vi "PhotonCamera_TakeOutputSnapshot.vi"(9 "BaseNTName":string="/photonvision", 11 "CameraName":string) -> (0 "error out":errorcluster)   [LabVIEW 2019, in "PhotonVisionLib.lvlib"]
doc: "Request the camera to save a new image file from the output stream with overlays. Images take up space in the filesystem of the PhotonCamera. Calling it frequently will fill up disk space and eventually cause the system to stop working. Clear out images in /opt/photonvision/photonvision_config/imgSaves frequently to prevent issues.\n\nInputs:\n - CameraName -- The nickname of the camera (found in the PhotonVision UI).\n - BaseNTName - string - Base Nework Table name. (Optional. Default: /photonvision )\n\nOutputs:\n - Error Out -- Contains error information if a Network table ot other error occured."
uses:
  PhotonVisionLib.lvlib
  <vilib>/Rock Robotics/WPI/ThirdParty/JAS_Junk/TrajLib/VI/Util_GetTime_U32.vi
  <vilib>/Rock Robotics/WPI/ThirdParty/JAS_Junk/TrajLib/VI/Util_GetTime_U64.vi
  <vilib>/Rock Robotics/Network Tables/NT Read Integer.vi
  <vilib>/Rock Robotics/Network Tables/NT Write Integer.vi
  <vilib>/Rock Robotics/WPI/ThirdParty/JAS_Junk/TrajLib/Trajectory_Library.lvlib
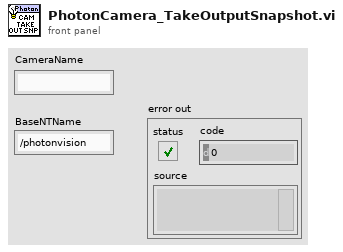
[diagram p1: front panel]
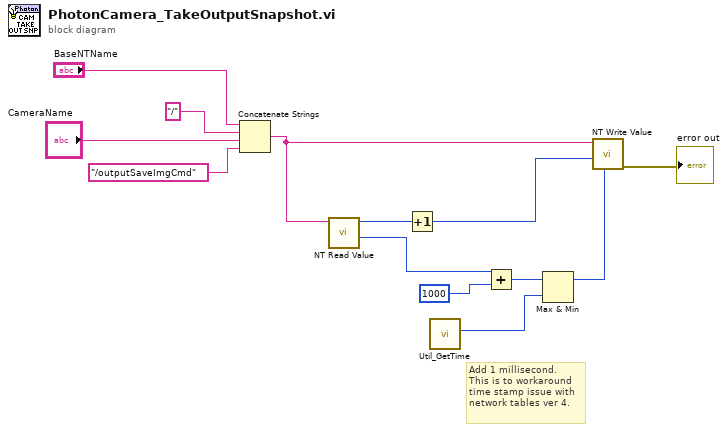
[diagram p0: block diagram]
diagram:
  # "Add 1 millisecond.\nThis is to workaround\ntime stamp issue with\nnetwork tables ver 4."
  n1 = Concatenate Strings("BaseNTName", "/" ("string"), "CameraName", "/outputSaveImgCmd") -> (w4:string)
  n2 = call-poly <vilib>:"NT Read Value.vi"("name"=w4) -> ("timestamp"=w6:u64, "value"=w11:i64)  [unwired: 8 in, 1 out]
  n3 = Increment(x=w11) -> (x+1=w10:i64)
  n4 = call <vilib>:"Util_GetTime.vi"() -> ("FPGA_Time_MicroSeconds"=w7:u64)  [unwired: 9 in, 2 out]
  n5 = Add(x=w6, y=u64 1000) -> (x+y=w8:u64)
  n6 = Max & Min(x=w8, y=w7) -> (max(x,y)=w5:u64)  [unwired: 1 out]
  n7 = call-poly <vilib>:"NT Write Value.vi"("timestamp"=w5, "value"=w10, "name"=w4) -> ("error out"=→"error out":errorcluster)  [unwired: 8 in]
